vi "RIMAS Detector SCP File From Server-v1.vi"(7 "Suffix data path":string, 8 "Error In":errorcluster, 10 "Detector Computer":T1={"Machine"="192.168.121.11", "Password"="rSL!nux12345", "FITS File Path"="/local/data/fermi-grb1/home/rimas/dev/h2rg/fitdat", "Port"=44444, "Header Path"="", "Name"=""}, 11 "Local file path":path=path "C:/Users/ZODI/Documents/LabVIEW Data/FITS Files") -> (0 "Error Out":errorcluster, 2 "log":string, 3 "Dup Local file path":path=path "C:/Users/ZODI/Documents/LabVIEW Data/FITS Files")   [LabVIEW 2024]
uses:
  RIMAS Detector Server Config.ctl
  <vilib>/Utility/error.llb/Trim Whitespace One-Sided.vi
panel:
  out "standard output":string
  out "cmd line":string
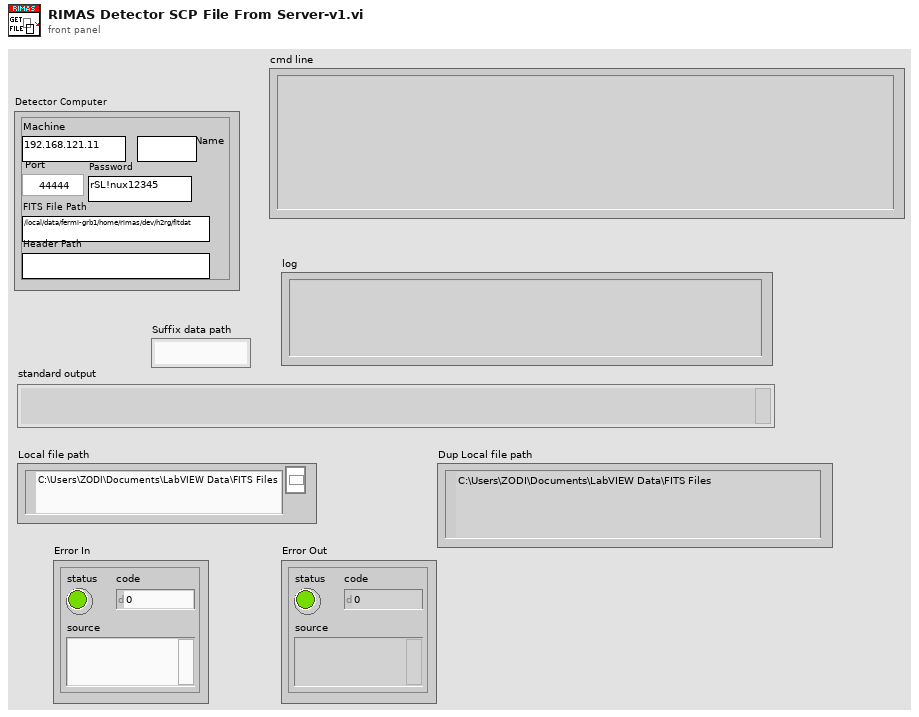
[diagram p1: front panel]
types:
  T1 = typedef "RIMAS Detector Server Config.ctl" = cluster{"Machine":string, "Password":string, "FITS File Path":string, "Port":u16, "Header Path":string, "Name":string}
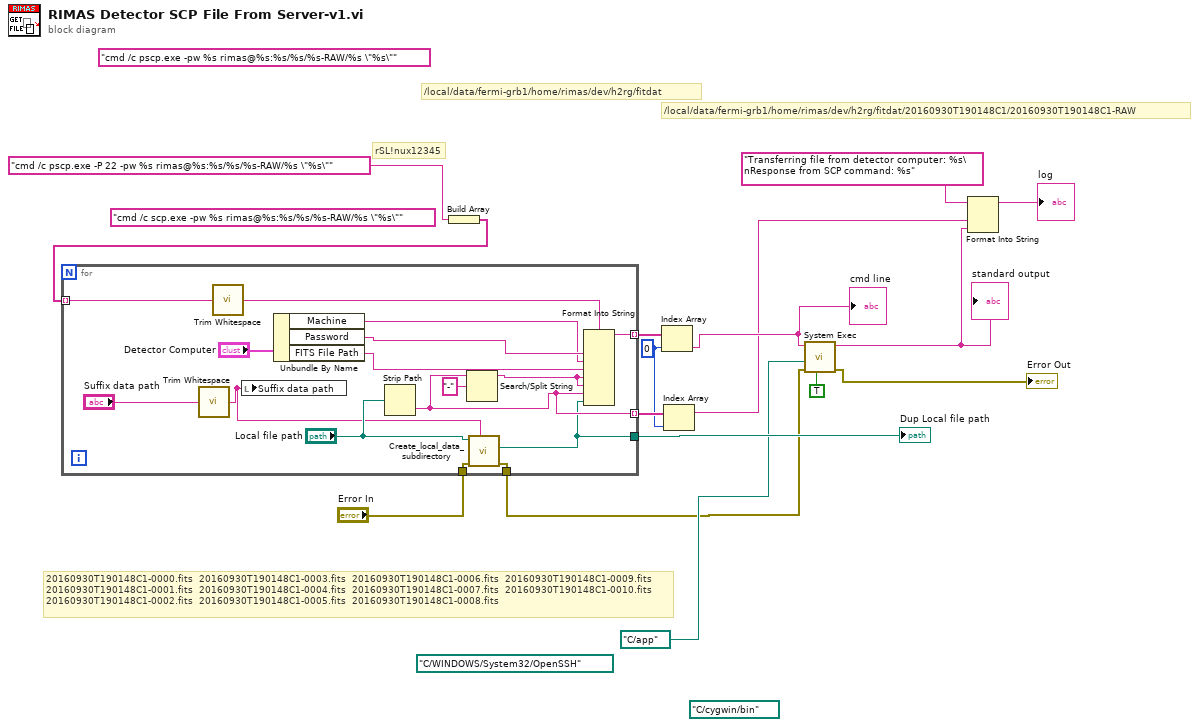
[diagram p0: block diagram]
diagram:
  (unwired) path "C:/WINDOWS/System32/OpenSSH" ("working directory")
  (unwired) "cmd /c scp.exe -pw %s rimas@%s:%s/%s/%s-RAW/%s \"%s\"" ("format string")
  w12 = 0 ("index")
  (unwired) path "C:/cygwin/bin" ("working directory")
  (unwired) "cmd /c pscp.exe -pw %s rimas@%s:%s/%s/%s-RAW/%s \"%s\"" ("format string")
  # "20160930T190148C1-0000.fits  20160930T190148C1-0003.fits  20160930T190148C1-0006.fits  20160930T190148C1-0009.fits\n20160930T190148C1-0001.fits  20160930T190148C1-0004.fits  20160930T190148C1-0007.fits  20160930T190148C1-0010.fits\n20160930T190148C1-0002.fits  20160930T190148C1-0005.fits  20160930T190148C1-0008.fits"
  # "/local/data/fermi-grb1/home/rimas/dev/h2rg/fitdat/20160930T190148C1/20160930T190148C1-RAW"
  # "/local/data/fermi-grb1/home/rimas/dev/h2rg/fitdat"
  # "rSL!nux12345"
  n1 = Build Array("cmd /c pscp.exe -P 22 -pw %s rimas@%s:%s/%s/%s-RAW/%s \"%s\"" ("format string")) -> (w9:string[])
  n2 = for {
    tunnel: [w32] -> w11 mode=indexing
    tunnel: [w25] -> w16 mode=indexing
    tunnel: [w19] -> w15
    tunnel: w9 -> [w24] mode=indexing
    tunnel: "Error In" -> [w21]
    tunnel: [w20] -> w7
    n3 = call <vilib>:"Trim Whitespace.vi"("string"="Suffix data path") -> ("trimmed string"=w17:string)  [unwired: 1 in]
    n4 = call <vilib>:"Trim Whitespace.vi"("string"=w24) -> ("trimmed string"=w23:string)  [unwired: 1 in]
    n5 = local write "Suffix data path"(w17) -> ()
    n6 = Unbundle By Name("Detector Computer") -> ("Machine"=w26:string, "Password"=w30:string, "FITS File Path"=w29:string)
    n7 = Strip Path(path="Local file path") -> (name=w25:string)  [unwired: 1 out]
    n8 = Search/Split String(string=w25, search string/char (-)="-") -> (substring before match=w27:string)  [unwired: 1 in, 2 out]
    n9 = call "Create_local_data_subdirectory.vi"("Suffix data path"=w17, "error in (no error)"=w21, "Local file path"="Local file path") -> ("error out"=w20:errorcluster, "Local file full path updated"=w19:path)  [unwired: 5 in, 2 out]
    n10 = Format Into String(format string=w23, w30, w26, w29, w27, w27, w25, w19) -> (resulting string=w32:string)  [unwired: 2 in, 1 out]
  }
  "Dup Local file path" <- w15
  n11 = Index Array(array=w11, index=w12) -> (element=w14:string)
  "cmd line" <- w14
  n12 = Index Array(array=w16, index=w12) -> (element=w13:string)
  n13 = call <vilib>:"System Exec.vi"("run minimized? (F)"=TRUE, "error in (no error)"=w7, "working directory"=path "C:/app", "command line"=w14) -> ("error out"=→"Error Out":errorcluster, "standard output"=w3:string)  [unwired: 4 in, 2 out]
  "standard output" <- w3
  n14 = Format Into String(format string="Transferring file from detector computer: %s\nResponse from SCP command: %s", w13, w3) -> (resulting string=→"log":string)  [unwired: 2 in, 1 out]
